vi "Destroy.vi"(11 "Circular Buffer in":refnum<class "Circular Buffer.lvclass">) -> ()   [LabVIEW 2021, in "d20.lvlib" / "Circular Buffer.lvclass"]
uses:
  Circular Buffer.lvclass
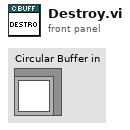
[diagram p1: front panel]
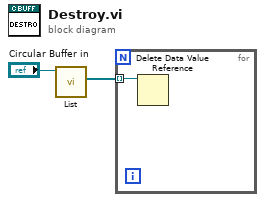
[diagram p0: block diagram]
diagram:
  n1 = call "List.vi"("Circular Buffer in"="Circular Buffer in") -> ("Node List"=w1:refnum<data-value>[])  [unwired: 7 in, 3 out]
  n2 = for {
    tunnel: w1 -> [w3] mode=indexing
    n3 = Delete Data Value Reference(data value reference=w3) -> ()  [unwired: 1 in, 2 out]
  }
